vi "DB Write ATR enable.vi"(0 "User ATR state Rx":u8, 1 "User input valid Rx":bool, 5 "stream session rx":refnum<class "niUSRP Stream Control (DMA) v1 FPGA.lvclass">, 9 "stream session tx":refnum<class "niUSRP Stream Control (DMA) v1 FPGA.lvclass">, 11 "User ATR state Tx":u8, 12 "User input valid Tx":bool) -> (4 "db 0":bool[](array[boolean]), 8 "db1":bool[](array[boolean]))   [LabVIEW 2025]
uses:
  Stream Control/niUSRP Stream Control (DMA) v1 FPGA.lvclass
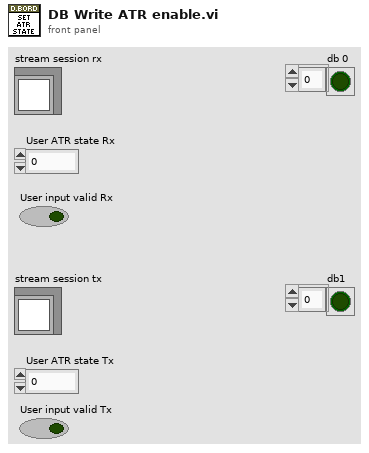
[diagram p1: front panel]
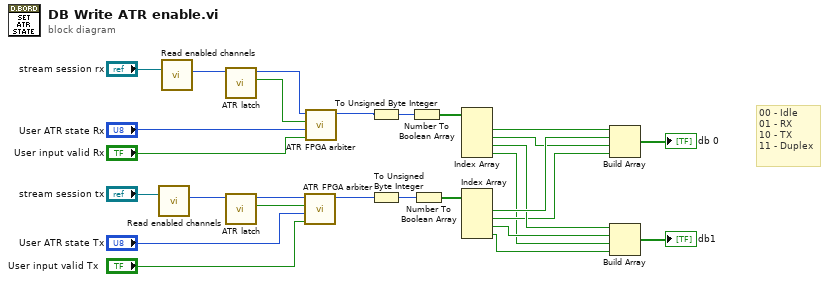
[diagram p0: block diagram]
diagram:
  # "00 - Idle \n01 - RX\n10 - TX\n11 - Duplex"
  n1 = call-dynamic "Read enabled channels.vi"("niUSRP Stream Control (DMA) v1 FPGA in"="stream session tx") -> ("enabled channels"=w5:u32)  [unwired: 9 in, 1 out]
  n2 = call-dynamic "Read enabled channels.vi"("niUSRP Stream Control (DMA) v1 FPGA in"="stream session rx") -> ("enabled channels"=w6:u32)  [unwired: 9 in, 1 out]
  n3 = call "ATR latch.vi"("enabled channels"=w6) -> ("new value"=w9:bool, "ATR  out"=w12:u8)  [unwired: 9 in]
  n4 = call "ATR latch.vi"("enabled channels"=w5) -> ("new value"=w10:bool, "ATR  out"=w11:u8)  [unwired: 9 in]
  n5 = call "ATR FPGA arbiter.vi"("User input valid"="User input valid Tx", "User ATR state"="User ATR state Tx", "RegBus input valid"=w10, "RegBus ATR state"=w11) -> ("ATR out"=w3:u8)  [unwired: 7 in]
  n6 = call "ATR FPGA arbiter.vi"("User input valid"="User input valid Rx", "User ATR state"="User ATR state Rx", "RegBus input valid"=w9, "RegBus ATR state"=w12) -> ("ATR out"=w4:u8)  [unwired: 7 in]
  n7 = To Unsigned Byte Integer(number=w4) -> (unsigned 8bit integer=w27:u8)
  n8 = To Unsigned Byte Integer(number=w3) -> (unsigned 8bit integer=w28:u8)
  n9 = Number To Boolean Array(number=w27) -> (Boolean array=w20:bool[])
  n10 = Number To Boolean Array(number=w28) -> (Boolean array=w19:bool[])
  n11 = Index Array(array=w20) -> (element #1=w24:bool, element #2=w17:bool, element #3=w22:bool, element #4=w15:bool)  [unwired: 4 in]
  n12 = Index Array(array=w19) -> (element #1=w23:bool, element #2=w16:bool, element #3=w21:bool, element #4=w14:bool)  [unwired: 4 in]
  n13 = Build Array(w24, w23, w17, w16) -> (→"db 0":bool[])
  n14 = Build Array(w22, w21, w15, w14) -> (→"db1":bool[])
